vi "DriveDistanceSubVi.vi"(4 "navX Device":T5 {"Interface"."Update Rate (4Hz-60Hz)" min=4 max=60 step=1}, 5 "EncoderDevRefLeft":T1, 6 "EncoderDevRefRight":T1, 7 "Setpoint":dbl, 8 "Angle":dbl, 9 "Deadband":dbl, 10 "VDeadband":dbl, 11 "Speed":dbl) -> (3 "Boolean":bool)   [LabVIEW 2015]
uses:
  NavX/navX Library v2/TypeDefs/Z900_navX_DeviceTypeDef.ctl
  NavX/navX Library v2/TypeDefs/Z900_navX_ProtocolTypeDef.ctl
  NavX/navX Library v2/TypeDefs/Z900_navX_NotifyPacketTypeDef.ctl
  NavX/navX Library v2/TypeDefs/Z900_navX_ActionTypeDef.ctl
  <vilib>/Rock Robotics/WPI/Encoder/WPI_EncoderDevRef.ctl
  <vilib>/Rock Robotics/SystemInterfaces/Encoder/FPGA_EncoderIdx.ctl
  <vilib>/Rock Robotics/SystemInterfaces/Counter/FPGA_CounterCtrSystemIndex.ctl
  <vilib>/Rock Robotics/WPI/Encoder/WPI_EncoderType.ctl
  <vilib>/Rock Robotics/Network Tables/NT Read Number.vi
  <vilib>/addons/control/pid/pid.llb/PID (DBL).vi
  <vilib>/addons/control/pid/NI_PID_pid.lvlib
  NavX/navX Library v2/navX Library v2.lvlib
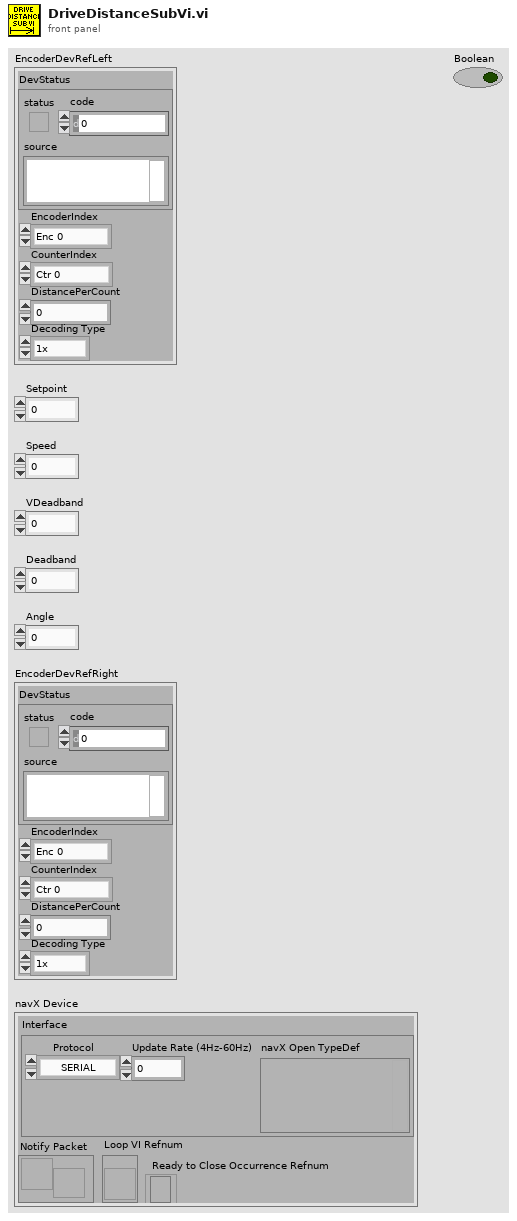
[diagram p1: front panel]
types:
  T1 = typedef "WPI_EncoderDevRef.ctl" = cluster{"DevStatus":errorcluster, "EncoderIndex":T2, "CounterIndex":T3, "DistancePerCount":dbl, "Decoding Type":T4}
  T2 = typedef "FPGA_EncoderIdx.ctl" = enum8{"Enc 0", "Enc 1", "Enc 2", "Enc 3", "Enc 4", "Enc 5", "Enc 6", "Enc 7", "Invalid"}
  T3 = typedef "FPGA_CounterCtrSystemIndex.ctl" = enum8{"Ctr 0", "Ctr 1", "Ctr 2", "Ctr 3", "Ctr 4", "Ctr 5", "Ctr 6", "Ctr 7", "Invalid"}
  T4 = typedef "WPI_EncoderType.ctl" = enum16{"1x", "2x", "4x"}
  T5 = typedef "navX Library v2.lvlib/Z900_navX_DeviceTypeDef.ctl" = cluster{"Interface":cluster{"Protocol":T6, "Update Rate (4Hz-60Hz)":u8, "navX Open TypeDef":variant}, "Notify Packet":refnum<notifier>, "Loop VI Refnum":refnum<vi>, "Ready to Close Occurrence Refnum":refnum<k4>}
  T6 = typedef "navX Library v2.lvlib/Z900_navX_ProtocolTypeDef.ctl" = enum16{"SERIAL", "I2C", "SPI"}
  T7 = cluster{"Numeric":dbl, "Numeric":dbl, "Numeric":dbl}
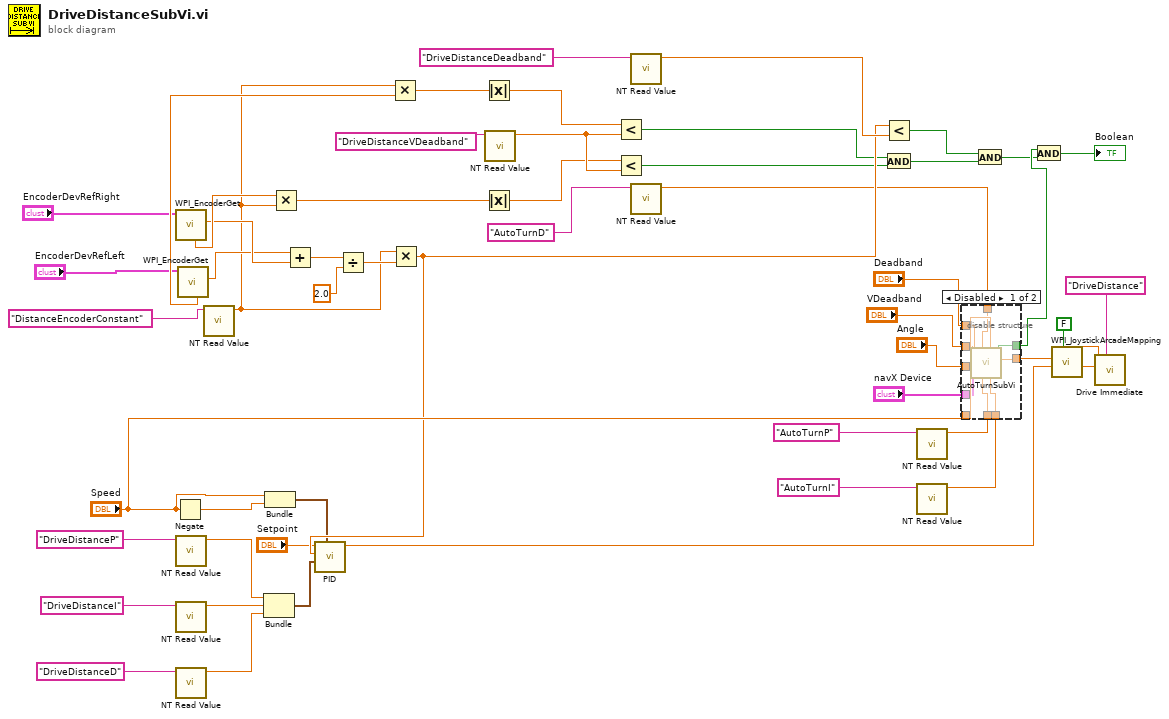
[diagram p0: block diagram]
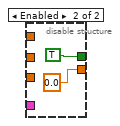
[diagram p2: hidden frame]
diagram:
  n1 = Negate(x="Speed") -> (-x=w13:dbl)
  n2 = call <vilib>:"WPI_EncoderGet.vi"("EncoderDevRef"="EncoderDevRefRight") -> ("Distance"=w8:dbl, "Rate"=w40:dbl)  [unwired: 5 in, 4 out]
  n3 = call-poly <vilib>:"NT Read Value.vi"("Name"="DriveDistanceP") -> ("Numeric"=w31:dbl)  [unwired: 9 in, 1 out]
  n4 = call-poly <vilib>:"NT Read Value.vi"("Name"="DriveDistanceI") -> ("Numeric"=w30:dbl)  [unwired: 9 in, 1 out]
  n5 = call-poly <vilib>:"NT Read Value.vi"("Name"="DriveDistanceD") -> ("Numeric"=w29:dbl)  [unwired: 9 in, 1 out]
  n6 = call <vilib>:"WPI_EncoderGet.vi"("EncoderDevRef"="EncoderDevRefLeft") -> ("Distance"=w7:dbl, "Rate"=w42:dbl)  [unwired: 5 in, 4 out]
  n7 = call-poly <vilib>:"NT Read Value.vi"("Name"="DistanceEncoderConstant") -> ("Numeric"=w2:dbl)  [unwired: 9 in, 1 out]
  n8 = Bundle("Numeric"=w31, "Numeric"=w30, "Numeric"=w29) -> (w15:T7)  [unwired: 1 in]
  n9 = Bundle("Speed"="Speed", w13) -> (w14:cluster{"Speed":dbl, dbl})  [unwired: 1 in]
  n10 = Multiply(x=w40, y=w2) -> (x*y=w39:dbl)
  n11 = Add(x=w7, y=w8) -> (x+y=w9:dbl)
  n12 = Divide(x=w9, y=2.0) -> (x/y=w11:dbl)
  n13 = Multiply(x=w2, y=w42) -> (x*y=w41:dbl)
  n14 = Multiply(x=w2, y=w11) -> (x*y=w43:dbl)
  n15 = call-poly <vilib>:"PID.vi"("output range"=w14, "PID gains"=w15, "process variable"=w43, "setpoint"="Setpoint") -> ("output"=w50:dbl)  [unwired: 6 in, 1 out]
  n16 = Absolute Value(x=w41) -> (abs(x)=w48:dbl)
  n17 = Absolute Value(x=w39) -> (abs(x)=w47:dbl)
  n18 = call-poly <vilib>:"NT Read Value.vi"("Name"="DriveDistanceVDeadband") -> ("Numeric"=w49:dbl)  [unwired: 9 in, 1 out]
  n19 = Less?(x=w48, y=w49) -> (x < y?=w37:bool)
  n20 = Less?(x=w47, y=w49) -> (x < y?=w38:bool)
  n21 = call-poly <vilib>:"NT Read Value.vi"("Name"="DriveDistanceDeadband") -> ("Numeric"=w44:dbl)  [unwired: 9 in, 1 out]
  n22 = call-poly <vilib>:"NT Read Value.vi"("Name"="AutoTurnD") -> ("Numeric"=w23:dbl)  [unwired: 9 in, 1 out]
  n23 = Less?(x=w43, y=w44) -> (x < y?=w46:bool)
  n24 = And(x=w37, y=w38) -> (x .and. y?=w45:bool)
  n25 = call-poly <vilib>:"NT Read Value.vi"("Name"="AutoTurnP") -> ("Numeric"=w25:dbl)  [unwired: 9 in, 1 out]
  n26 = call-poly <vilib>:"NT Read Value.vi"("Name"="AutoTurnI") -> ("Numeric"=w24:dbl)  [unwired: 9 in, 1 out]
  n27 = disable-structure shown="Disabled" {
    disable-tunnel: [w64 TRUE ("Boolean")] -> w53
    disable-tunnel: "Speed" -> [w63 _]
    disable-tunnel: "Angle" -> [w62 _]
    disable-tunnel: "Deadband" -> [w61 _]
    disable-tunnel: "VDeadband" -> [w60 _]
    disable-tunnel: w25 -> [w59 _]
    disable-tunnel: w24 -> [w58 _]
    disable-tunnel: w23 -> [w57 _]
    disable-tunnel: "navX Device" -> [w56 _]
    disable-tunnel: [w55 0.0 ("X axis value")] -> w1
    frame Disabled {
      n28 = call "AutoTurnSubVi.vi"("I"=w58, "Speed"=w63, "P"=w59, "D"=w57, "navX Device"=w56, "Angle"=w62, "VDeadband"=w60, "Deadband"=w61) -> ("Output"=w55:dbl, "Boolean"=w64:bool)  [unwired: 2 in]
    }
    frame Enabled {
    }
  }
  n29 = And(x=w46, y=w45) -> (x .and. y?=w52:bool)
  n30 = And(x=w53, y=w52) -> (x .and. y?=→"Boolean":bool)
  n31 = call <vilib>:"WPI_JoystickArcadeMapping.vi"("Square Inputs"=FALSE, "Y axis value"=w50, "X axis value"=w1) -> ("Right Motor Value"=w17:dbl, "Left Motor Value"=w16:dbl)  [unwired: 7 in]
  n32 = call "Drive Immediate.vi"("Description"="DriveDistance", "Right Setpoint"=w17, "Left Setpoint"=w16) -> ()  [unwired: 8 in, 1 out]
